vi "Read NVMEMArea.Size.vi"(8 "error in (no error)":errorcluster, 11 "SLSC Remote in":refnum<class "SLSC Remote.lvclass">) -> (0 "error out":errorcluster, 2 "NVMEMArea.Size":u32, 3 "SLSC Remote out":refnum<class "SLSC Remote.lvclass">)   [LabVIEW 2015, in "SLSC Remote.lvclass"]
uses:
  SLSC Remote.lvclass
  SLSC Interface Class/SLSC Interface.lvclass
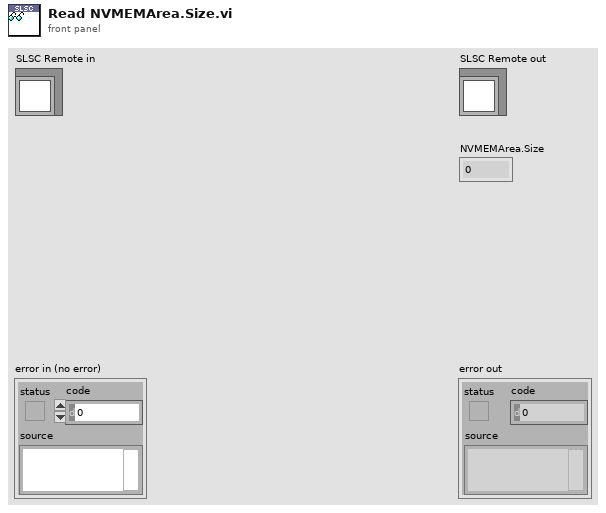
[diagram p1: front panel]
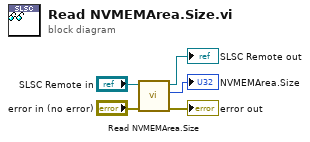
[diagram p0: block diagram]
diagram:
  n1 = call-parent "Read NVMEMArea.Size.vi"("error in (no error)"="error in (no error)", "SLSC Interface in"="SLSC Remote in") -> ("error out"=→"error out":errorcluster, "NVMEMArea.Size"=→"NVMEMArea.Size":u32, "SLSC Interface out"=→"SLSC Remote out":refnum<class "SLSC Remote.lvclass">)  [unwired: 7 in]
